vi "数值到十六进制字符串.vi"(10 "Numeric":u32=23, 11 "转换字节数":enum16{"1字节", "2字节", "4字节", "3字节"}(ring)) -> (3 "转换结果":string)   [LabVIEW 2013]
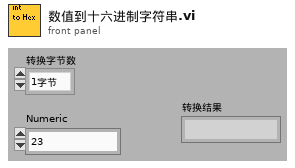
[diagram p1: front panel]
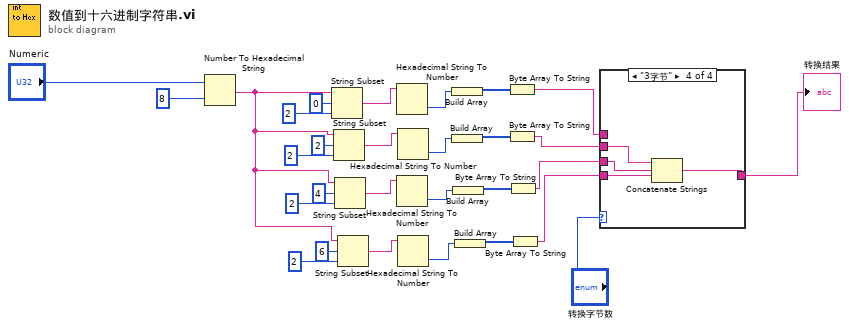
[diagram p0: block diagram]
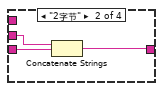
[diagram p3: hidden frame]
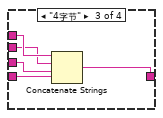
[diagram p4: hidden frame]
diagram:
  n1 = Number To Hexadecimal String(1:i16 8 ("width (-)"), 2:"Numeric") -> (0:w20:string)
  n2 = String Subset(string=w20, offset (0)=0, length (rest)=2 ("length (rest)")) -> (substring=w19:string)
  n3 = String Subset(string=w20, offset (0)=2, length (rest)=2 ("length (rest)")) -> (substring=w18:string)
  n4 = String Subset(string=w20, offset (0)=4, length (rest)=2 ("length (rest)")) -> (substring=w17:string)
  n5 = String Subset(string=w20, offset (0)=6, length (rest)=2 ("length (rest)")) -> (substring=w16:string)
  n6 = Hexadecimal String To Number(string=w19) -> (number=w11:u32)  [unwired: 3 out]
  n7 = Hexadecimal String To Number(string=w17) -> (number=w9:u32)  [unwired: 3 out]
  n8 = Hexadecimal String To Number(string=w18) -> (number=w10:u32)  [unwired: 3 out]
  n9 = Hexadecimal String To Number(string=w16) -> (number=w8:u32)  [unwired: 3 out]
  n10 = Build Array(w11) -> (w15:u32[])
  n11 = Build Array(w10) -> (w14:u32[])
  n12 = Build Array(w9) -> (w13:u32[])
  n13 = Build Array(w8) -> (w12:u32[])
  n14 = Byte Array To String(unsigned byte array=w15) -> (string=w1:string)
  n15 = Byte Array To String(unsigned byte array=w14) -> (string=w2:string)
  n16 = Byte Array To String(unsigned byte array=w13) -> (string=w3:string)
  n17 = Byte Array To String(unsigned byte array=w12) -> (string=w4:string)
  n18 = case shown="\"3字节\"" "转换字节数" {
    tunnel: [w30 w31 w36 w40] -> w5
    tunnel: w4 -> [w30 w33 w38 w42]
    tunnel: w3 -> [_ w32 w37 w41]
    tunnel: w2 -> [_ _ w34 w39]
    tunnel: w1 -> [_ _ w35 _]
    frame "1字节", Default {
    }
    frame "2字节" {
      n19 = Concatenate Strings(w32, w33) -> (w31:string)
    }
    frame "4字节" {
      n20 = Concatenate Strings(w35, w34, w37, w38) -> (w36:string)
    }
    frame "3字节" {
      n21 = Concatenate Strings(w39, w41, w42) -> (w40:string)
    }
  }
  "转换结果" <- w5
